vi "DSF.Engine.Memory.Transfer.Get ID.vi"(8 "error in (no error)":errorcluster, 11 "Transfer in":refnum<class "DSF.Engine.Memory.Transfer.lvclass">) -> (0 "error out":errorcluster, 2 "id":i32, 3 "Transfer out":refnum<class "DSF.Engine.Memory.Transfer.lvclass">)   [LabVIEW 2016, in "DSF.Engine.lvlib" / "DSF.Engine.Memory.Transfer.lvclass"]
uses:
  DSF.Engine.Memory.Transfer.lvclass
  DSF.Engine.Memory.Transfer.lvclass/DSF.Engine.Memory.Transfer.ctl
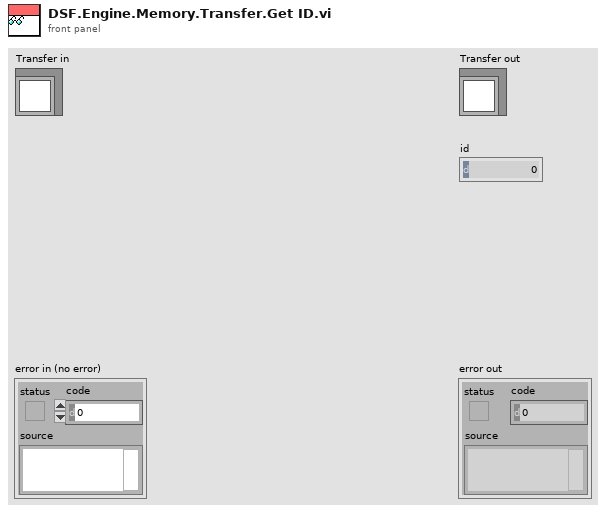
[diagram p1: front panel]
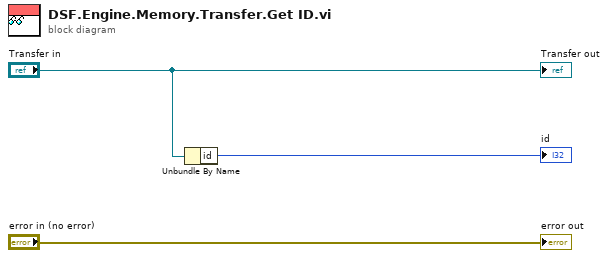
[diagram p0: block diagram]
diagram:
  n1 = Unbundle By Name("Transfer in") -> ("id"=→"id":i32)
  "error out" <- "error in (no error)"
  "Transfer out" <- "Transfer in"
